vi "Get MB Registers.vi"(8 "error in (no error)":errorcluster, 10 "Register Names":string[](array[string]), 11 "HPS17K IP Address":string) -> (0 "error out":errorcluster, 3 "Register Data":string[][](array[string]))   [LabVIEW 2023, in "HPS-17000-PowerModule.lvlib" / "HPS-17000-PowerModule.lvclass"]
uses:
  HPS-17000-PowerModule.lvclass
  <vilib>/net/SSH/Client/PuTTY/PuTTY Client.lvclass
  C:/Program Files/National Instruments/LabVIEW 2023/vi.lib/net/SSH/Client/Generic/Generic Client.lvclass
  <vilib>/net/SSH/Client/Generic/Generic Client.lvclass/Generic Client.ctl
  <vilib>/net/SSH/Client/Generic/Write trust on first use.vi
  <vilib>/Utility/error.llb/Trim Whitespace One-Sided.vi
  HPS-17000-PowerModule.lvclass/HPS-17000-PowerModule.ctl
  <vilib>/net/SSH/NI_SSH.lvlib
  C:/Program Files/National Instruments/LabVIEW 2023/vi.lib/net/SSH/Client/PuTTY/PuTTY Client.lvclass
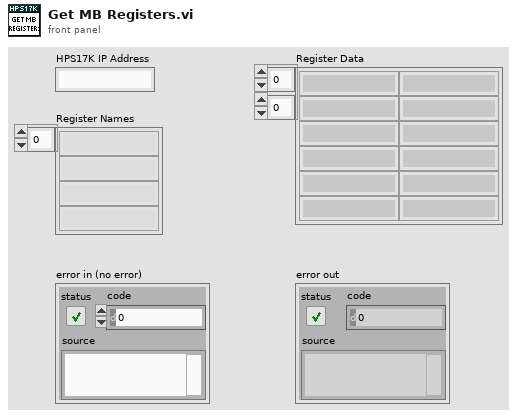
[diagram p1: front panel]
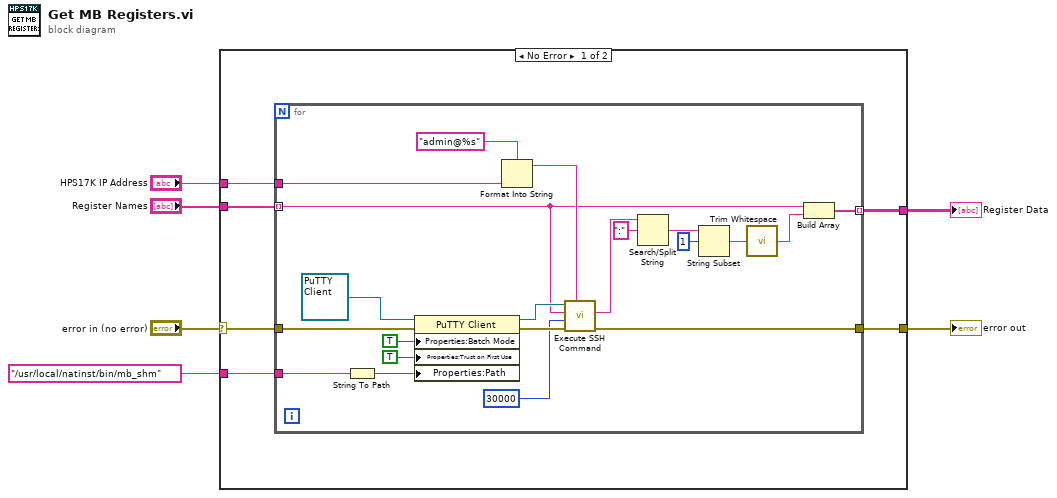
[diagram p0: block diagram]
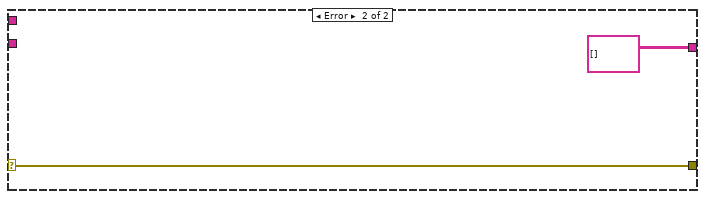
[diagram p2: hidden frame]
diagram:
  n1 = case shown="No Error" "error in (no error)" {
    selector: "error in (no error)" -> [w7 w35]
    tunnel: "HPS17K IP Address" -> [w12 _]
    tunnel: "/usr/local/natinst/bin/mb_shm" -> [w11 _]
    tunnel: "Register Names" -> [w10 _]
    tunnel: [w9 string[][] []] -> w3
    tunnel: [w8 w35] -> w2
    frame No Error {
      n2 = for {
        tunnel: w7 -> [w18]
        tunnel: [w17] -> w8
        tunnel: w10 -> [w14] mode=indexing
        tunnel: [w28] -> w9 mode=indexing
        tunnel: w11 -> [w15]
        tunnel: w12 -> [w13]
        n3 = String To Path(string=w15) -> (path=w24:path)
        n4 = property class="PuTTY Client"(reference=refnum<class "PuTTY Client.lvclass"> refnum ("NI_SSH.lvlib:PuTTY Client"), error in=w18, "Properties:Batch Mode"=TRUE ("Batch Mode"), "Properties:Trust on First Use"=TRUE ("Trust on First Use"), "Properties:Path"=w24) -> (reference out=w26:refnum<class "PuTTY Client.lvclass">, error out=w25:errorcluster)
        n5 = Format Into String(format string="admin@%s", w13) -> (resulting string=w27:string)  [unwired: 2 in, 1 out]
        n6 = call <vilib>:"Execute SSH Command.vi"("user@host"=w27, "error in (no error)"=w25, "timeout (ms)"=30000, "command line"=w14, "session in"=w26) -> ("error out"=w17:errorcluster, "standard output"=w16:string)  [unwired: 2 in, 3 out]
        n7 = Search/Split String(string=w16, search string/char (-)=":") -> (match + rest of string=w31:string)  [unwired: 1 in, 2 out]
        n8 = String Subset(string=w31, offset (0)=1) -> (substring=w30:string)  [unwired: 1 in]
        n9 = call <vilib>:"Trim Whitespace.vi"("string"=w30) -> ("trimmed string"=w29:string)  [unwired: 1 in]
        n10 = Build Array(w14, w29) -> (w28:string[])
      }
    }
    frame Error {
    }
  }
  "Register Data" <- w3
  "error out" <- w2
